vi "VI Tree.vi"   [LabVIEW 2013, in "Agilent E364X Series.lvlib"]
doc: "Displays all the VI of the instrument driver in an organized table."
uses:
  <instrlib>/Agilent E364X Series/Agilent E364X Series.lvlib
panel:
  # "© 2005 National Instruments.  ALL RIGHTS RESERVED."
  # "See Diagram Box\nfor VI Tree"
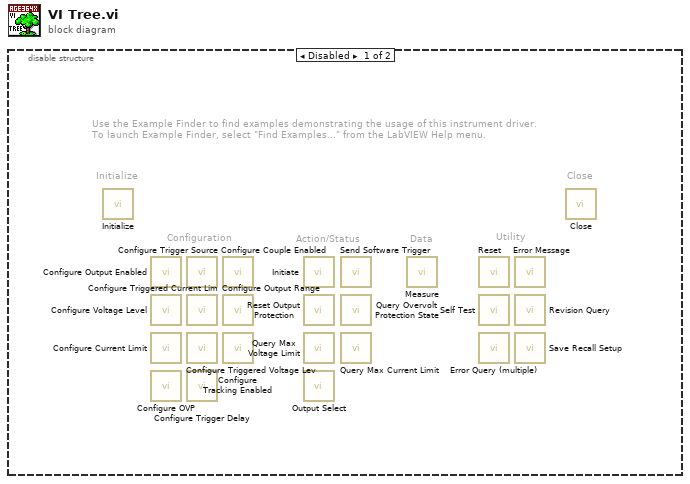
[diagram p0: block diagram]
diagram:
  n1 = disable-structure shown="Disabled" {
    frame Disabled {
      # "Use the Example Finder to find examples demonstrating the usage of this instrument driver.\nTo launch Example Finder, select \"Find Examples...\" from the LabVIEW Help menu."
      # "Close"
      # "Utility"
      # "Data"
      # "Action/Status"
      # "Configuration"
      # "Initialize"
      n2 = call <instrlib>:"Initialize.vi"() -> ()  [unwired: 10 in, 2 out]
      n3 = call <instrlib>:"Configure Output Enabled.vi"() -> ()  [unwired: 10 in, 2 out]
      n4 = call <instrlib>:"Configure Voltage Level.vi"() -> ()  [unwired: 10 in, 2 out]
      n5 = call <instrlib>:"Configure Current Limit.vi"() -> ()  [unwired: 10 in, 2 out]
      n6 = call <instrlib>:"Configure OVP.vi"() -> ()  [unwired: 10 in, 2 out]
      n7 = call <instrlib>:"Configure Trigger Source.vi"() -> ()  [unwired: 10 in, 2 out]
      n8 = call <instrlib>:"Configure Triggered Current Lim.vi"() -> ()  [unwired: 10 in, 2 out]
      n9 = call <instrlib>:"Configure Triggered Voltage Lev.vi"() -> ()  [unwired: 10 in, 2 out]
      n10 = call <instrlib>:"Configure Trigger Delay.vi"() -> ()  [unwired: 10 in, 2 out]
      n11 = call <instrlib>:"Configure Couple Enabled.vi"() -> ()  [unwired: 10 in, 2 out]
      n12 = call <instrlib>:"Configure Output Range.vi"() -> ()  [unwired: 10 in, 2 out]
      n13 = call <instrlib>:"Configure Tracking Enabled.vi"() -> ()  [unwired: 10 in, 2 out]
      n14 = call <instrlib>:"Initiate.vi"() -> ()  [unwired: 10 in, 2 out]
      n15 = call <instrlib>:"Reset Output Protection.vi"() -> ()  [unwired: 10 in, 2 out]
      n16 = call <instrlib>:"Query Max Voltage Limit.vi"() -> ()  [unwired: 9 in, 3 out]
      n17 = call <instrlib>:"Output Select.vi"() -> ()  [unwired: 10 in, 2 out]
      n18 = call <instrlib>:"Send Software Trigger.vi"() -> ()  [unwired: 10 in, 2 out]
      n19 = call <instrlib>:"Query Overvolt Protection State.vi"() -> ()  [unwired: 9 in, 3 out]
      n20 = call <instrlib>:"Query Max Current Limit.vi"() -> ()  [unwired: 9 in, 3 out]
      n21 = call <instrlib>:"Measure.vi"() -> ()  [unwired: 9 in, 3 out]
      n22 = call <instrlib>:"Reset.vi"() -> ()  [unwired: 10 in, 2 out]
      n23 = call <instrlib>:"Self Test.vi"() -> ()  [unwired: 8 in, 4 out]
      n24 = call <instrlib>:"Error Query (multiple).vi"() -> ()  [unwired: 8 in, 4 out]
      n25 = call <instrlib>:"Error Message.vi"() -> ()  [unwired: 11 in, 5 out]
      n26 = call <instrlib>:"Revision Query.vi"() -> ()  [unwired: 8 in, 4 out]
      n27 = call <instrlib>:"Save Recall Setup.vi"() -> ()  [unwired: 10 in, 2 out]
      n28 = call <instrlib>:"Close.vi"() -> ()  [unwired: 11 in, 1 out]
    }
    frame Enabled {
    }
  }
